vi "Close File.vi"(8 "error in":errorcluster, 11 "Refnum":refnum<file>) -> (0 "error out":errorcluster, 3 "UTF-8 Path":refnum<class "UTF-8 Path.lvclass">)   [LabVIEW 2020, in "G-Unicode.lvlib"]
doc: "Closes an open file specified by <b>Refnum</b> and returns the UTF-8 path to the file associated with the refnum."
uses:
  G-Unicode.lvlib
  Types/UTF-8 Path/UTF-8 Path.lvclass
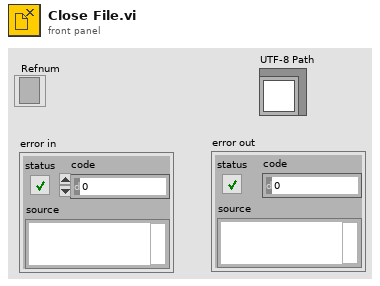
[diagram p1: front panel]
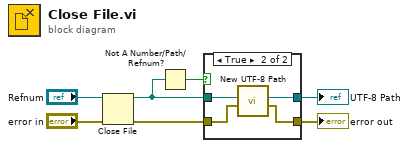
[diagram p0: block diagram]
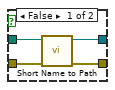
[diagram p2: hidden frame]
diagram:
  n1 = Close File(refnum="Refnum", error in="error in") -> (path=w3:path, error out=w2:errorcluster)
  n2 = Not A Number/Path/Refnum?(number/path/refnum=w3) -> (NaN/Path/Refnum?=w1:bool)
  n3 = case shown="True" w1 {
    tunnel: w3 -> [w11 w15]
    tunnel: [w8 w14] -> w5
    tunnel: [w10 w12] -> w4
    tunnel: w2 -> [w9 w13]
    frame False {
      n4 = call "Short Name to Path.vi"("error in"=w9, "LabVIEW Path"=w11) -> ("error out"=w10:errorcluster, "UTF-8 Path"=w8:refnum<class "UTF-8 Path.lvclass">)  [unwired: 8 in]
    }
    frame True {
      n5 = call "New UTF-8 Path.vi"("error in"=w13, "LabVIEW Path"=w15) -> ("error out"=w12:errorcluster, "UTF-8 Path"=w14:refnum<class "UTF-8 Path.lvclass">)  [unwired: 8 in]
    }
  }
  "UTF-8 Path" <- w5
  "error out" <- w4
